vi "Write Default channels.vi"(8 "error in (no error)":errorcluster, 10 "Default channels":string[][](array[string]), 11 "MagLabGraph in":refnum<class "MagLabGraph.lvclass">) -> (0 "error out":errorcluster, 3 "MagLabGraph out":refnum<class "MagLabGraph.lvclass">)   [LabVIEW 2015, in "MagLabGraph.lvclass"]
uses:
  MagLabGraph.lvclass
  MagLabGraph.lvclass/MagLabGraph.ctl
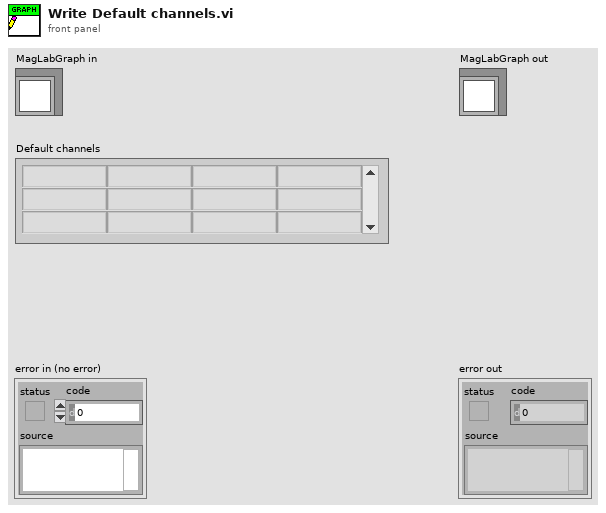
[diagram p1: front panel]
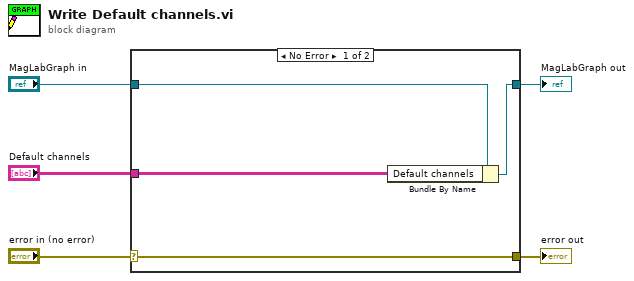
[diagram p0: block diagram]
diagram:
  n1 = case shown="No Error" "error in (no error)" {
    selector: "error in (no error)" -> [w9 w10]
    tunnel: [w9 w10] -> w4
    tunnel: [w7 w11] -> w2
    tunnel: "MagLabGraph in" -> [w8 w11]
    tunnel: "Default channels" -> [w6 _]
    frame No Error {
      n2 = Bundle By Name(cluster=w8, "Default channels"=w6) -> (w7:refnum<class "MagLabGraph.lvclass">)
    }
    frame Error {
    }
  }
  "error out" <- w4
  "MagLabGraph out" <- w2
